vi "ScanDelayFindResource.vi"(8 "error in (no error)":errorcluster, 11 "Remote Host (none)":string) -> (0 "error out":errorcluster, 2 "return count":u32, 3 "resource array":string[](array[string]))   [LabVIEW 2018]
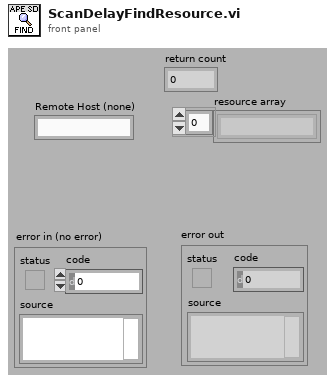
[diagram p1: front panel]
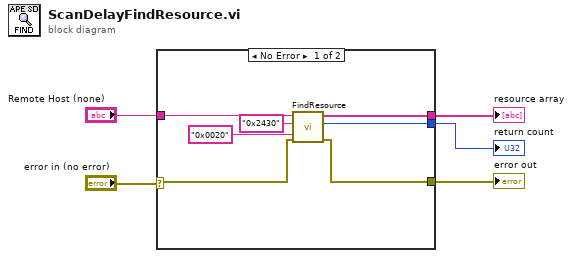
[diagram p0: block diagram]
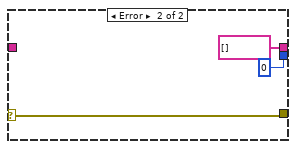
[diagram p2: hidden frame]
diagram:
  n1 = case shown="No Error" "error in (no error)" {
    selector: "error in (no error)" -> [w6 w15]
    tunnel: "Remote Host (none)" -> [w12 _]
    tunnel: [w9 string[] [] ("resource array")] -> w2
    tunnel: [w8 w15] -> w3
    tunnel: [w7 u32 0 ("return count")] -> w1
    frame No Error {
      n2 = call "FindResource.vi"("error in (no error)"=w6, "Product ID"="0x0020", "Vendor ID"="0x2430", "Remote Host (none)"=w12) -> ("error out"=w8:errorcluster, "return count"=w7:u32, "resource array"=w9:string[])  [unwired: 5 in]
    }
    frame Error {
    }
  }
  "error out" <- w3
  "resource array" <- w2
  "return count" <- w1
